vi "GetValue.vi"(8 "error in":errorcluster, 11 "IntergerMeasure in":refnum<class "IntegerMeasure.lvclass">) -> (0 "error out":errorcluster, 2 "Value":i64, 3 "IntergerMeasure out":refnum<class "IntegerMeasure.lvclass">)   [LabVIEW 2021, in "ProligentXMLGenerator.lvlib" / "IntegerMeasure.lvclass"]
doc: "Defines the value acquired by the measure."
uses:
  IntegerMeasure.lvclass
  IntegerMeasure.lvclass/IntegerMeasure.ctl
  Base/Integer/Integer.lvclass
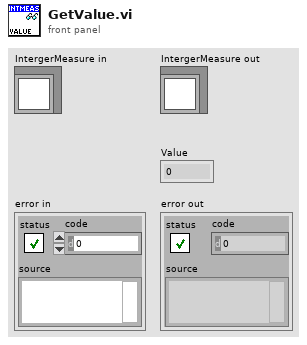
[diagram p1: front panel]
types:
  T1 = typedef "ProligentXMLGenerator.lvlib/IntegerMeasure.lvclass/Data.ctl" = cluster{"Value":refnum<class "Integer.lvclass">}
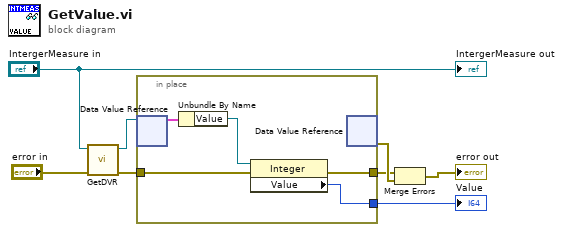
[diagram p0: block diagram]
diagram:
  n1 = call "GetDVR.vi"("error in"="error in", "IntergerMeasure"="IntergerMeasure in") -> ("error out"=w4:errorcluster, "DVRReference"=w3:refnum<data-value>)  [unwired: 8 in]
  n2 = in-place "In Place Element Structure" {
    in-place-border: [w9] -> w2
    in-place-border: w4 -> [w11]
    in-place-border: [w10] -> w5
    n3 = in-place-dvr #1(w3) -> (w13:T1)  [unwired: 1 out]
    n4 = Unbundle By Name(w13) -> ("Value"=w12:refnum<class "Integer.lvclass">)
    n5 = property class="Integer"(reference=w12, error in=w11) -> (error out=w10:errorcluster, "Value"=w9:i64)  [unwired: 1 out]
    n6 = in-place-dvr #1() -> (w6:errorcluster)  [unwired: 1 in, 1 out]
  }
  "Value" <- w2
  n7 = Merge Errors(w5, w6) -> (→"error out":errorcluster)
  "IntergerMeasure out" <- "IntergerMeasure in"
